vi "CRYGet Property in Graph.vi"(11 "Graph VI Ref":refnum<vi>) -> (3 "Flattened Property":string)   [LabVIEW 2013]
uses:
  Control/CRYResult Property.ctl
  Control/CRYTable Property.ctl
  Control/CRYPicture Property.ctl
  Control/CRYText Property.ctl
  Control/CRYPolar Property.ctl
  Control/CRYIntensity Property.ctl
panel:
  in  "Intensity Property":T1={"Time Steps"=0, "Frequency Bins"=0, "Type"=0, "Length"=0, "Map Type"=enum."rainbow"} {"Type" items=["Rectangle"=0, "Hanning"=1, "Hamming"=2, "Blackman-Harris"=3, "Exact Blackman"=4, "Blackman"=5, "Flat Top"=6, "4 Term B-Harris"=7, "7 Term B-Harris"=8, "Low Sidelobe"=9, "Blackman Nuttall"=11, "Triangle"=30, "Bartlett-Hanning"=31, "Bohman"=32, "Parzen"=33, "Welch"=34, "Kaiser"=60, "Dolph-Chebyshev"=61, "Gaussian"=62]}
  in  "Polar Property":T2={"polar attributes"={"maximum"=2.0, "minimum"=0.0, "clip to min"=FALSE, "log"=FALSE, "grid color"=3381657, "plot color"=16711680, "fmt and prec"={"format"=enum."Decimal", "precision"=2}, "visible section"=4}, "Auto/Manual"=0, "Zero Adjust (deg)"=0, "Angle Increment (deg)"=0, "Mirror"=FALSE, "Auto Increment"=FALSE, "Total Rotatin (deg)"=0, "Discrete/Rannge"=0, "Show Name"=FALSE, "CurValues"=[], "CurIndex"=0, "CurColors"=[], "CurColors_Range"=[], "CurValues_Range"=[], "Pen"={"Width"=1, "Style"=enum."Solid"}, "BackgroundColor"=0} {"polar attributes"."minimum" format="%0.2f"; "polar attributes"."maximum" format="%0.2f"}
  in  "Text Format":T3
  in  "Picture Property":T4
  in  "Table Property":T5 {"Precision" items=["Digits of precision", "Significant digits"]}
  in  "Result Property":T6={"Show Limits"=FALSE, "Show Yield"=FALSE, "Pass/Fail"=FALSE, "Notation"=0, "Digits"=0, "Precision"=0, "Hide Traling Zeros"=FALSE, "Show vertical scroll bar"=FALSE, "Show horizontal scroll bar"=FALSE, "True"="NO ELECTRICAL SIGNAL DETECTED!\nCheck wiring and connections.", "False"="NO ELECTRICAL SIGNAL DETECTED!\nCheck wiring and connections.", "Font Size"=0, "Overall/Optional"=0} {"Precision" items=["Digits of precision", "Significant digits"]}
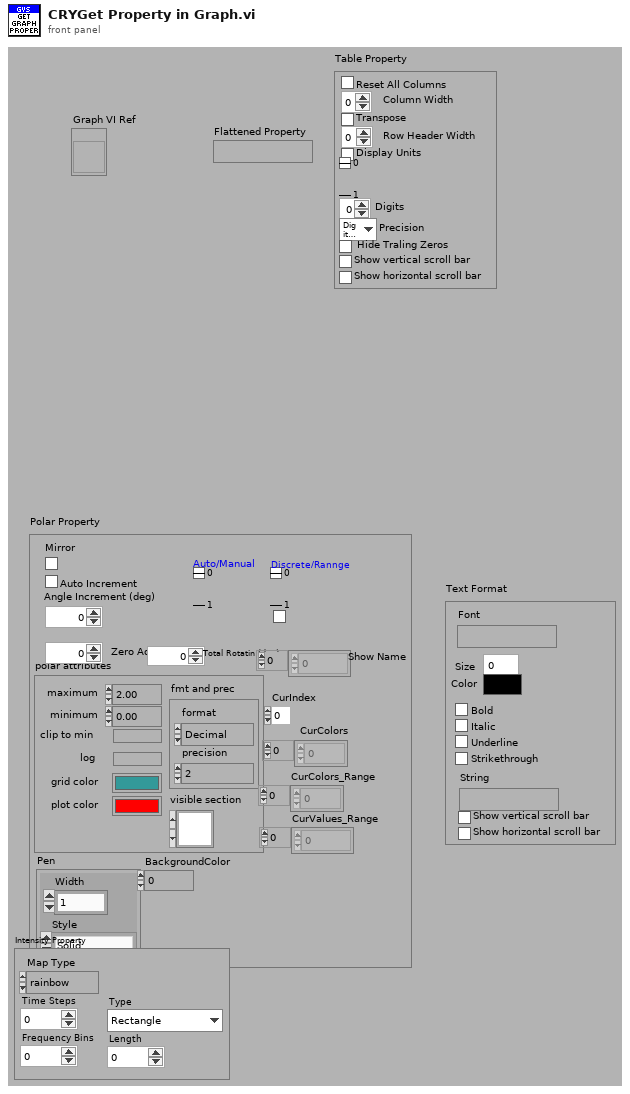
[diagram p1: front panel]
types:
  T1 = typedef "CRYIntensity Property.ctl" = cluster{"Time Steps":i32, "Frequency Bins":i32, "Type":u32, "Length":i32, "Map Type":enum16{"fire", "rainbow", "grey", "inverse grey", "ice", "original"}}
  T2 = typedef "CRYPolar Property.ctl" = cluster{"polar attributes":cluster{"maximum":dbl, "minimum":dbl, "clip to min":bool, "log":bool, "grid color":u32, "plot color":u32, "fmt and prec":cluster{"format":enum8{"Decimal", "Scientific", "Engineering", "Binary", "Octal", "Hex"}, "precision":u8}, "visible section":u16}, "Auto/Manual":u16, "Zero Adjust (deg)":i32, "Angle Increment (deg)":i32, "Mirror":bool, "Auto Increment":bool, "Total Rotatin (deg)":i32, "Discrete/Rannge":u16, "Show Name":bool, "CurValues":dbl[], "CurIndex":u16, "CurColors":u32[], "CurColors_Range":u32[], "CurValues_Range":dbl[], "Pen":cluster{"Width":u16, "Style":enum32{"Solid", "Dash", "Dot", "DashDot", "DashDotDot"}}, "BackgroundColor":u32}
  T3 = typedef "CRYText Property.ctl" = cluster{"Size":u32, "Bold":bool, "Italic":bool, "Underline":bool, "Strikethrough":bool, "Color":u32, "Font":string, "String":string, "Show vertical scroll bar":bool, "Show horizontal scroll bar":bool}
  T4 = typedef "CRYPicture Property.ctl" = cluster{"Image Path":string, "Show vertical scroll bar":bool, "Show horizontal scroll bar":bool}
  T5 = typedef "CRYTable Property.ctl" = cluster{"Reset All Columns":bool, "Transpose":bool, "Display Units":bool, "Notation":u16, "Digits":u16, "Precision":u16, "Hide Traling Zeros":bool, "Column Width":u16, "Row Header Width":u16, "Show vertical scroll bar":bool, "Show horizontal scroll bar":bool}
  T6 = typedef "CRYResult Property.ctl" = cluster{"Show Limits":bool, "Show Yield":bool, "Pass/Fail":bool, "Notation":u16, "Digits":u16, "Precision":u16, "Hide Traling Zeros":bool, "Show vertical scroll bar":bool, "Show horizontal scroll bar":bool, "True":string, "False":string, "Font Size":u16, "Overall/Optional":u16}
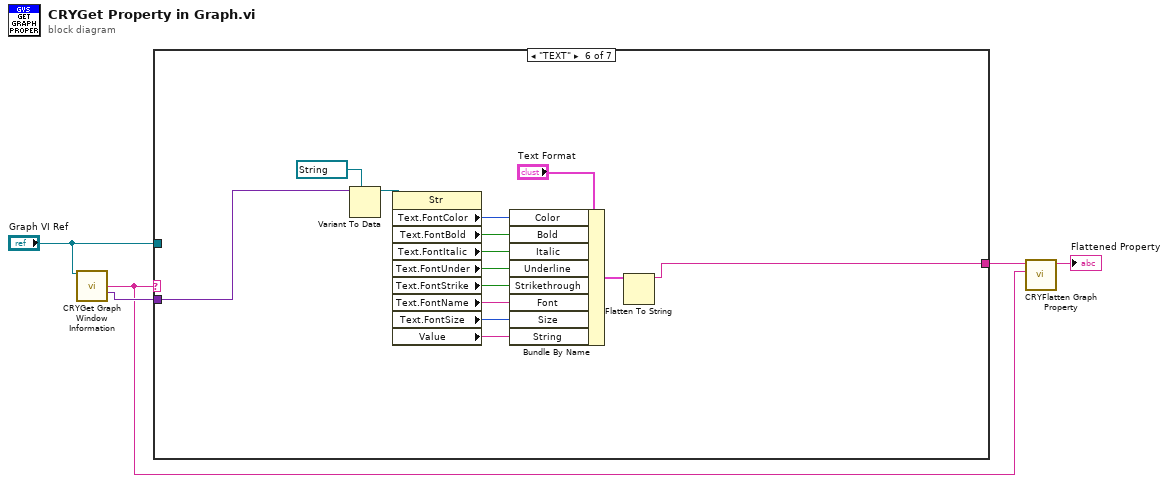
[diagram p0: block diagram]
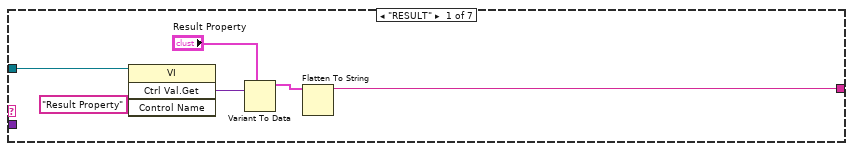
[diagram p2: hidden frame]
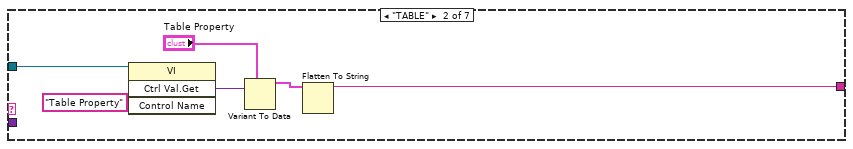
[diagram p3: hidden frame]
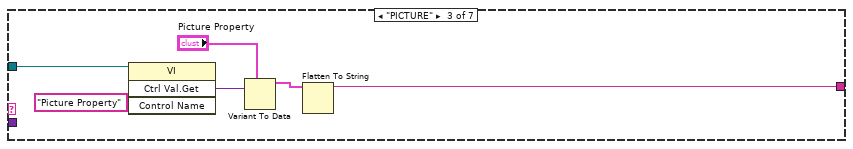
[diagram p4: hidden frame]
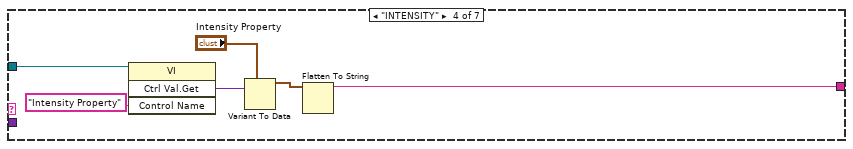
[diagram p5: hidden frame]
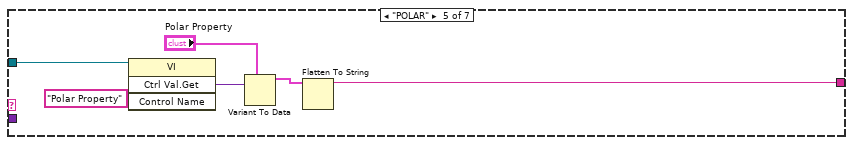
[diagram p6: hidden frame]
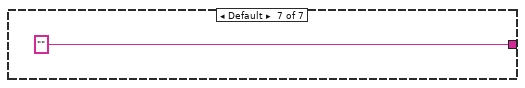
[diagram p7: hidden frame]
diagram:
  n1 = call "CRYGet Graph Window Information.vi"("pGraph VI In"="Graph VI Ref") -> ("Graph Type Out"=w1:string, "Graph Control Ref Out"=w4:variant)  [unwired: 4 in, 9 out]
  n2 = case shown="\"TEXT\"" w1 {
    tunnel: [w6 w14 w20 w26 w32 w36 "" ("data string")] -> w3
    tunnel: "Graph VI Ref" -> [w7 w13 w19 w25 w31 _ _]
    tunnel: w4 -> [_ _ _ _ _ w38 _]
    frame "RESULT" {
      n3 = invoke class="VI" method="Ctrl Val.Get"(reference=w7, "Control Name"="Result Property") -> ("Get Control Value Variant"=w10:variant)  [unwired: 2 in, 3 out]
      n4 = Variant To Data(type="Result Property", Variant=w10) -> (data=w8:T6)  [unwired: 1 in, 1 out]
      n5 = Flatten To String(anything=w8) -> (data string=w6:string)  [unwired: 3 in, 2 out]
    }
    frame "TABLE" {
      n6 = invoke class="VI" method="Ctrl Val.Get"(reference=w13, "Control Name"="Table Property") -> ("Get Control Value Variant"=w16:variant)  [unwired: 2 in, 3 out]
      n7 = Variant To Data(type="Table Property", Variant=w16) -> (data=w15:T5)  [unwired: 1 in, 1 out]
      n8 = Flatten To String(anything=w15) -> (data string=w14:string)  [unwired: 3 in, 2 out]
    }
    frame "PICTURE" {
      n9 = invoke class="VI" method="Ctrl Val.Get"(reference=w19, "Control Name"="Picture Property") -> ("Get Control Value Variant"=w22:variant)  [unwired: 2 in, 3 out]
      n10 = Variant To Data(type="Picture Property", Variant=w22) -> (data=w21:T4)  [unwired: 1 in, 1 out]
      n11 = Flatten To String(anything=w21) -> (data string=w20:string)  [unwired: 3 in, 2 out]
    }
    frame "INTENSITY" {
      n12 = invoke class="VI" method="Ctrl Val.Get"(reference=w25, "Control Name"="Intensity Property") -> ("Get Control Value Variant"=w28:variant)  [unwired: 2 in, 3 out]
      n13 = Variant To Data(type="Intensity Property", Variant=w28) -> (data=w27:T1)  [unwired: 1 in, 1 out]
      n14 = Flatten To String(anything=w27) -> (data string=w26:string)  [unwired: 3 in, 2 out]
    }
    frame "POLAR" {
      n15 = invoke class="VI" method="Ctrl Val.Get"(reference=w31, "Control Name"="Polar Property") -> ("Get Control Value Variant"=w34:variant)  [unwired: 2 in, 3 out]
      n16 = Variant To Data(type="Polar Property", Variant=w34) -> (data=w33:T2)  [unwired: 1 in, 1 out]
      n17 = Flatten To String(anything=w33) -> (data string=w32:string)  [unwired: 3 in, 2 out]
    }
    frame "TEXT" {
      n18 = Variant To Data(type=refnum<vi> refnum ("Graph Ref"), Variant=w38) -> (data=w49:refnum<vi>)  [unwired: 1 in, 1 out]
      n19 = property class="Str"(reference=w49) -> ("Text.FontColor"=w48:u32, "Text.FontBold"=w47:bool, "Text.FontItalic"=w46:bool, "Text.FontUnder"=w45:bool, "Text.FontStrike"=w44:bool, "Text.FontName"=w43:string, "Text.FontSize"=w42:u32, "Value"=w41:string)  [unwired: 1 in, 2 out]
      n20 = Bundle By Name(cluster="Text Format", "Color"=w48, "Bold"=w47, "Italic"=w46, "Underline"=w45, "Strikethrough"=w44, "Font"=w43, "Size"=w42, "String"=w41) -> (w40:T3)
      n21 = Flatten To String(anything=w40) -> (data string=w36:string)  [unwired: 3 in, 2 out]
    }
    frame Default {
    }
  }
  n22 = call "CRYFlatten Graph Property.vi"("Cluster Name"=w1, "GraphProperty"=w3) -> ("GraphProperty Flattened"=→"Flattened Property":string)  [unwired: 9 in]
